vi "test-swerve-drve-kinematics-ALL.vi"(8 "error in (no error)":errorcluster) -> (0 "error out":errorcluster, 3 "ALL TEsts Passed":bool)   [LabVIEW 2019]
panel:
  out "Test 17":bool
  out "Test 16":bool
  out "Test 15":bool
  out "Test 14":bool
  out "Test 13":bool
  out "Test 12":bool
  out "Test 11":bool
  out "Test 10":bool
  out "Test 9":bool
  out "Test 8":bool
  out "Test 7":bool
  out "Test 6":bool
  out "Test 5":bool
  out "Test 4":bool
  out "Test 3":bool
  out "Test 2":bool
  out "Test 1":bool
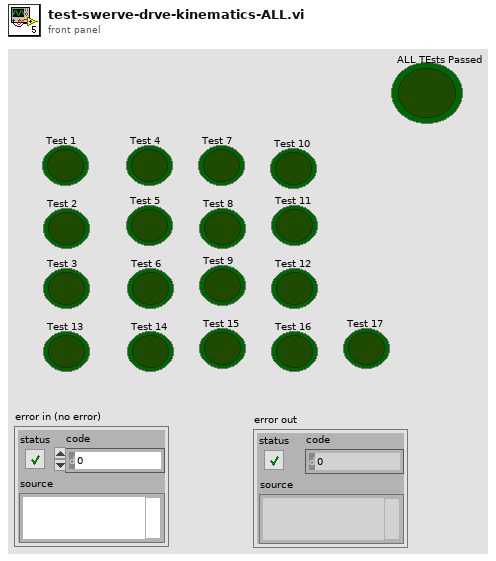
[diagram p1: front panel]
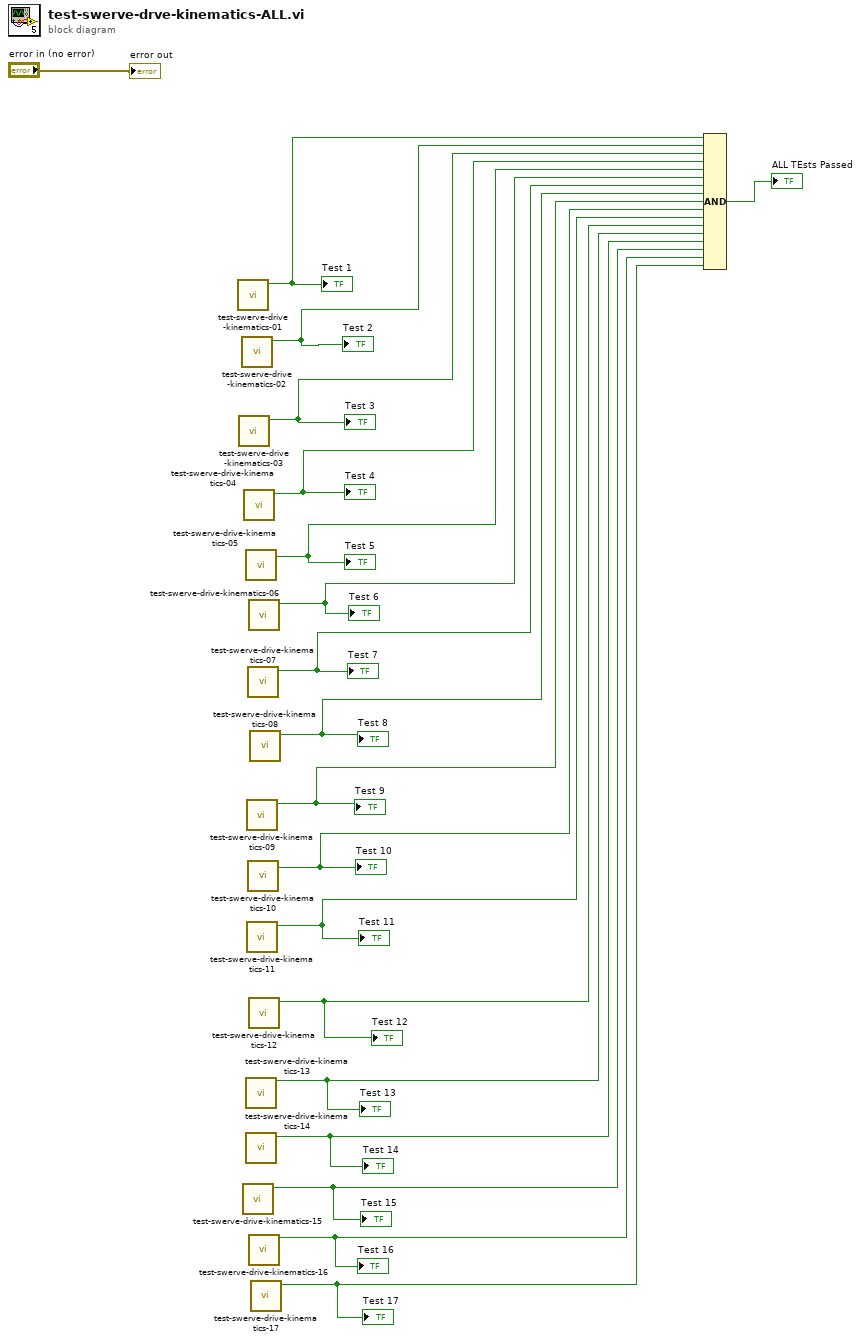
[diagram p0: block diagram]
diagram:
  n1 = call "test-swerve-drive-kinematics-01.vi"() -> ("Test Passed"=w17:bool)  [unwired: 11 in]
  "Test 1" <- w17
  n2 = call "test-swerve-drive-kinematics-03.vi"() -> ("Test Passed"=w15:bool)  [unwired: 11 in]
  "Test 3" <- w15
  n3 = call "test-swerve-drive-kinematics-02.vi"() -> ("Test Passed"=w16:bool)  [unwired: 11 in]
  "Test 2" <- w16
  n4 = call "test-swerve-drive-kinematics-15.vi"() -> ("Test Passed"=w3:bool)  [unwired: 11 in]
  "Test 15" <- w3
  n5 = call "test-swerve-drive-kinematics-04.vi"() -> ("Test Passed"=w14:bool)  [unwired: 11 in]
  "Test 4" <- w14
  n6 = call "test-swerve-drive-kinematics-05.vi"() -> ("Test Passed"=w13:bool)  [unwired: 11 in]
  "Test 5" <- w13
  n7 = call "test-swerve-drive-kinematics-13.vi"() -> ("Test Passed"=w5:bool)  [unwired: 11 in]
  "Test 13" <- w5
  n8 = call "test-swerve-drive-kinematics-14.vi"() -> ("Test Passed"=w4:bool)  [unwired: 11 in]
  "Test 14" <- w4
  n9 = call "test-swerve-drive-kinematics-09.vi"() -> ("Test Passed"=w9:bool)  [unwired: 11 in]
  "Test 9" <- w9
  n10 = call "test-swerve-drive-kinematics-11.vi"() -> ("Test Passed"=w7:bool)  [unwired: 11 in]
  "Test 11" <- w7
  n11 = call "test-swerve-drive-kinematics-07.vi"() -> ("Test Passed"=w11:bool)  [unwired: 11 in]
  "Test 7" <- w11
  n12 = call "test-swerve-drive-kinematics-10.vi"() -> ("Test Passed"=w8:bool)  [unwired: 11 in]
  "Test 10" <- w8
  n13 = call "test-swerve-drive-kinematics-06.vi"() -> ("Test Passed"=w12:bool)  [unwired: 11 in]
  "Test 6" <- w12
  n14 = call "test-swerve-drive-kinematics-12.vi"() -> ("Test Passed"=w6:bool)  [unwired: 11 in]
  "Test 12" <- w6
  n15 = call "test-swerve-drive-kinematics-16.vi"() -> ("Test Passed"=w2:bool)  [unwired: 11 in]
  "Test 16" <- w2
  n16 = call "test-swerve-drive-kinematics-08.vi"() -> ("Test Passed"=w10:bool)  [unwired: 11 in]
  "Test 8" <- w10
  n17 = call "test-swerve-drive-kinematics-17.vi"() -> ("Test Passed"=w1:bool)  [unwired: 11 in]
  "Test 17" <- w1
  n18 = Compound Arithmetic op=AND(w17, w16, w15, w14, w13, w12, w11, w10, w9, w8, w7, w6, w5, w4, w3, w2, w1) -> (→"ALL TEsts Passed":bool)
  "error out" <- "error in (no error)"
